vi "Fetch All Operators.vi"(8 "error in (no error)":errorcluster, 10 "SQL Statement":string="SELECT ModelNumber FROM TestConfigurations", 11 "Database in":refnum<queue>) -> (0 "error out":errorcluster, 2 "Operators":string[](array[string]), 3 "Database out":refnum<queue>)   [LabVIEW 2026]
uses:
  support/Architecture/Message Queue/Message Queue.lvlib
  support/Architecture/Message Queue/Enqueue Message (Single).vi
  controls/Messaging Payloads/DB Query Request Payload.ctl
  controls/UI/UI List Type.ctl
  controls/UI/Measurement Role Selection.ctl
  Settings.lvlib
  controls/UI/Data Entity.ctl
  support/Architecture/Message Queue/Message Cluster.ctl
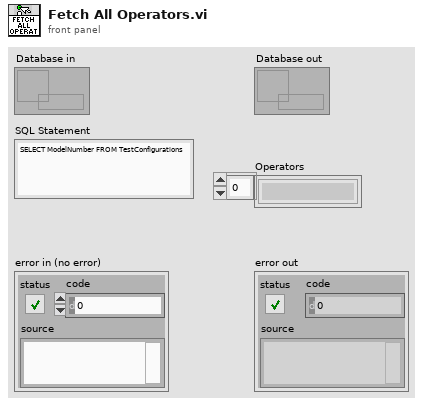
[diagram p1: front panel]
types:
  T1 = typedef "DB Query Request Payload.ctl" = cluster{"1D Notifier":refnum<notifier>, "UI List Type":T2, "UI Device Type":T3, "Identifier":i32, "2D Notifier":refnum<notifier>, "Measurement Role Selection":T4}
  T2 = typedef "UI List Type.ctl" = enum16{"Model Numbers", "Serial Numbers", "Operators", "Calibration Points", "Start Run Times"}
  T3 = typedef "Settings.lvlib/Data Entity.ctl" = enum16{"Measurement", "Controller", " Test Configuration"}
  T4 = typedef "Settings.lvlib/Measurement Role Selection.ctl" = enum16{"Controller", "Reference", "UUT", "All"}
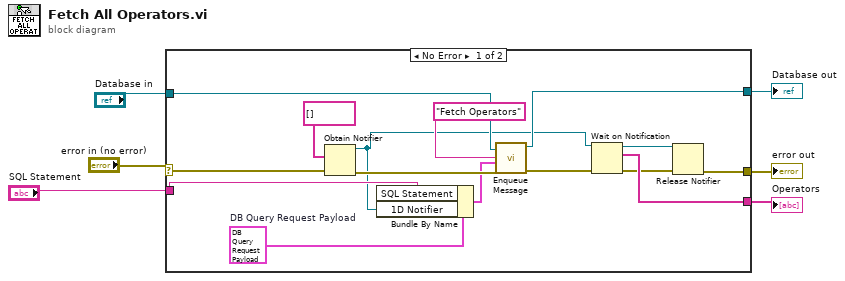
[diagram p0: block diagram]
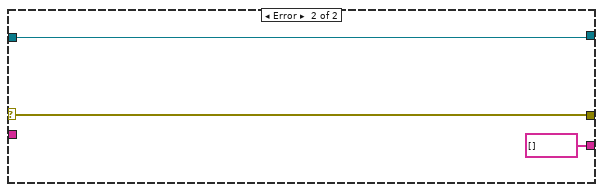
[diagram p2: hidden frame]
diagram:
  n1 = case shown="No Error" "error in (no error)" {
    selector: "error in (no error)" -> [w11 w23]
    tunnel: [w21 string[] []] -> w6
    tunnel: [w20 w24] -> w5
    tunnel: "Database in" -> [w19 w24]
    tunnel: [w18 w23] -> w3
    tunnel: "SQL Statement" -> [w9 _]
    frame No Error {
      w10 = T1 {"1D Notifier"=refnum, "UI List Type"=enum."Model Numbers", "UI Device Type"=enum."Measurement", "Identifier"=0, "2D Notifier"=refnum, "Measurement Role Selection"=enum."Controller"}  # DB Query Request Payload
      n2 = Obtain Notifier(notification data type=string[] [], error in (no error)=w11) -> (notifier out=w8:refnum<notifier>, error out=w14:errorcluster)  [unwired: 2 in, 1 out]
      n3 = Bundle By Name(cluster=w10, "SQL Statement"=w9, "1D Notifier"=w8) -> (w7:T1)
      n4 = call-poly "Enqueue Message.vi"("error in (no error)"=w14, "Message Data"=w7, "Message"="Fetch Operators", "Message Queue"=w19) -> ("error out"=w15:errorcluster, "dup Message Queue"=w20:refnum<queue>)  [unwired: 6 in]
      n5 = Wait on Notification(notifier=w8, error in (no error)=w15) -> (notifier out=w17:refnum<notifier>, notification=w21:string[], error out=w16:errorcluster)  [unwired: 2 in, 1 out]
      n6 = Release Notifier(notifier=w17, error in (no error)=w16) -> (error out=w18:errorcluster)  [unwired: 1 in, 2 out]
    }
    frame Error {
    }
  }
  "Operators" <- w6
  "Database out" <- w5
  "error out" <- w3
